vi "InitStringQueue.vi"(7 "StackMaxNumber":i32=-1, 8 "error in (no error)":errorcluster, 9 "QueueType":string, 11 "QueueName":string) -> (0 "error out":errorcluster, 3 "StackOut":variant)   [LabVIEW 2013]
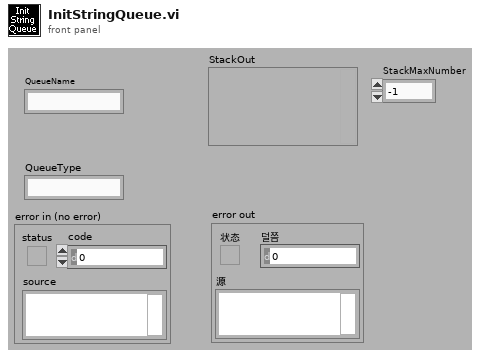
[diagram p1: front panel]
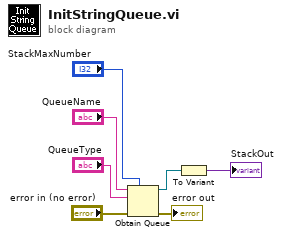
[diagram p0: block diagram]
diagram:
  n1 = Obtain Queue(max queue size (-1, unlimited)="StackMaxNumber", name (unnamed)="QueueName", element data type="QueueType", error in (no error)="error in (no error)") -> (queue out=w5:refnum<queue>, error out=→"error out":errorcluster)  [unwired: 1 in, 1 out]
  n2 = To Variant(anything=w5) -> (Variant=→"StackOut":variant)
